vi "Launch Update Project Wizard.vi"(8 "error in (no error)":errorcluster, 11 "Controller in":refnum<class "Controller.lvclass">) -> (0 "error out":errorcluster, 3 "Controller out":refnum<class "Controller.lvclass">)   [LabVIEW 2013, in "SET Project Editor.lvlib" / "Controller.lvclass"]
uses:
  Controller.lvclass
  Wizards/Update Project Wizard/Update Project Wizard.lvclass
  Controller.lvclass/Controller.ctl
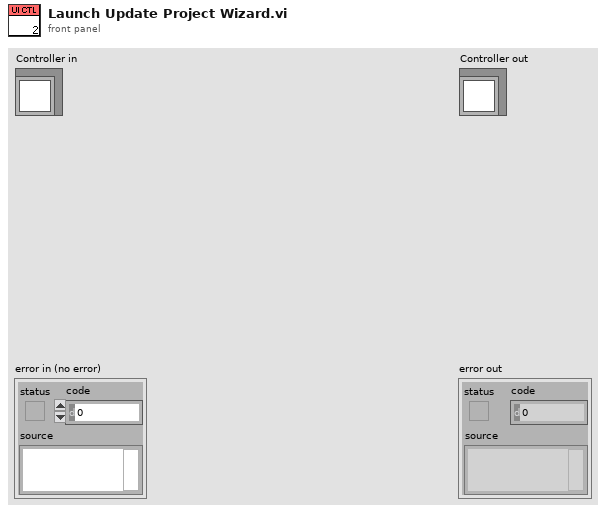
[diagram p1: front panel]
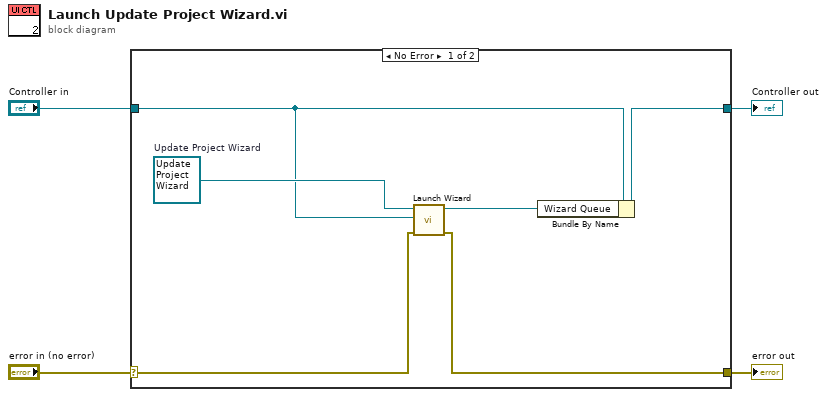
[diagram p0: block diagram]
diagram:
  n1 = case shown="No Error" "error in (no error)" {
    selector: "error in (no error)" -> [w9 w12]
    tunnel: [w8 w12] -> w3
    tunnel: [w5 w11] -> w1
    tunnel: "Controller in" -> [w6 w11]
    frame No Error {
      w10 = refnum<class "Update Project Wizard.lvclass"> refnum  # Update Project Wizard
      n2 = call-dynamic "Launch Wizard.vi"("error in (no error)"=w9, "Controller in"=w6, "New Project Wizard in"=w10) -> ("error out"=w8:errorcluster, "Caller-To-Actor Enqueuer"=w7:refnum<class "Message Enqueuer.lvclass">)  [unwired: 7 in]
      n3 = Bundle By Name(cluster=w6, "Wizard Queue"=w7) -> (w5:refnum<class "Controller.lvclass">)
    }
    frame Error {
    }
  }
  "error out" <- w3
  "Controller out" <- w1
